vi "Examples - AcquisitionTest.vi"() -> ()   [LabVIEW 2018]
panel:
  in  "Stop":bool
  out "Image":T1(plugin-control)
  # "Use this button instead of Abort Execution button"
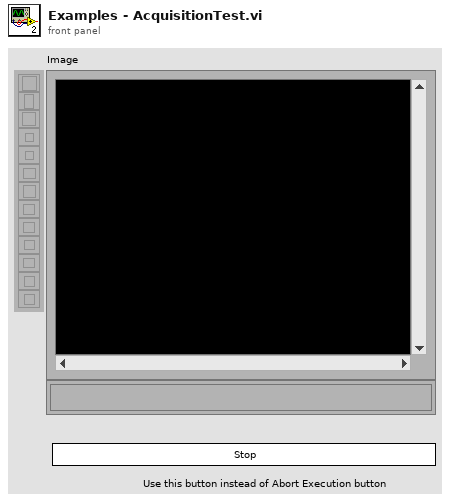
[diagram p1: front panel]
types:
  T1 = typedef "IMAQ Image.ctl" = refnum<image>
  T2 = typedef "Image Type" = u32
  T3 = typedef "xiImageMng - Attributes.ctl" = cluster{"WIDTH":i32, "HEIGHT":i32, "IMG_FORMAT":T4}
  T4 = typedef "IMG_DATA_FORMAT.ctl" = enum16{"MONO8", "MONO16", "RGB24", "RGB32", "RGBPLANAR", "RAW8", "RAW16"}
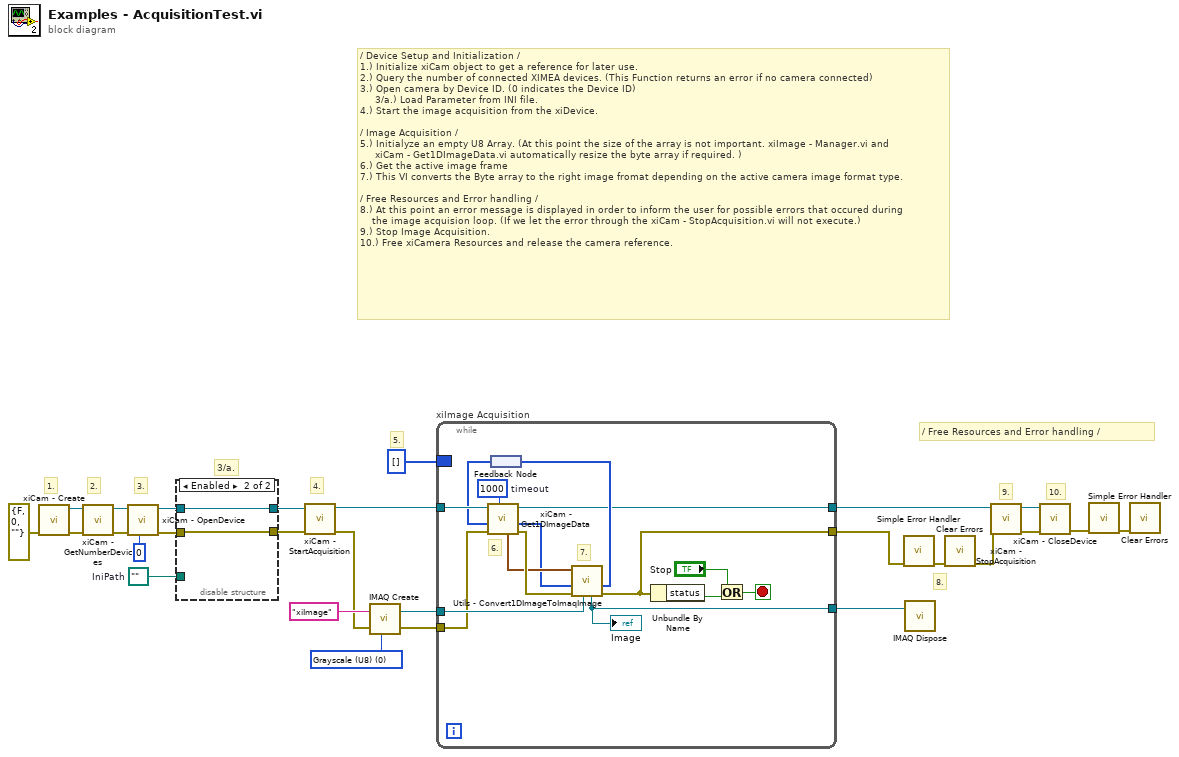
[diagram p0: block diagram]
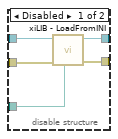
[diagram p2: hidden frame]
diagram:
  w4 = T2 0 items=["Grayscale (U8)", "Grayscale (I16)", "Grayscale (SGL)", "Complex (CSG)", "RGB (U32)", "HSL (U32)", "RGB (U64)", "Grayscale (U16)"] ("Image Type")
  w5 = path ""  # IniPath
  # "3/a."
  # "/ Free Resources and Error handling /"
  # "9."
  # "10."
  # "8."
  # "5."
  # "/ Device Setup and Initialization /\n1.) Initialize xiCam object to get a reference for later use.\n2.) Query the number of connected XIMEA devices. (This Function returns an error if no camera connected)\n3.) Open camera by Device ID. (0 indicates the Device ID)\n     3/a.) Load Parameter from INI file. \n4.) Start the image acquisition from the xiDevice.\n\n/ Image Acquisition /\n5.) Initialyze an empty U8 Array. (At this point the size of the array is not important. xiImage - Manager.vi and\n     xiCam - Get1DImageData.vi automatically resize the byte array if required. )\n6.) Get the active image frame\n7.) This VI converts the Byte array to the right image fromat depending on the active camera image format type.\n\n/ Free Resources and Error handling /\n8.) At this point an error message is displayed in order to inform the user for possible errors that occured during\n    the image acquision loop. (If we let the error through the xiCam - StopAcquisition.vi will not execute.)\n9.) Stop Image Acquisition.\n10.) Free xiCamera Resources and release the camera reference."
  # "4."
  # "3."
  # "2."
  # "1."
  n1 = call "xiCam - Create.vi"("error in (no error)"=errorcluster {"status"=FALSE, "code"=0, "source"=""}) -> ("error out"=w26:errorcluster, "new xiCam"=w27:refnum<k24>)  [unwired: 9 in]
  n2 = call "xiCam - GetNumberDevices.vi"("error in (no error)"=w26, "xiCam In"=w27) -> ("error out"=w24:errorcluster, "xiCam Out"=w25:refnum<k24>)  [unwired: 7 in, 1 out]
  n3 = call "xiCam - OpenDevice.vi"("DevID"=0, "error in (no error)"=w24, "xiCam In"=w25) -> ("error out"=w6:errorcluster, "xiCam Out"=w7:refnum<k24>)  [unwired: 7 in]
  n4 = disable-structure shown="Enabled" {
    disable-tunnel: w7 -> [w32 w34]
    disable-tunnel: [w31 w34] -> w3
    disable-tunnel: [w30 w33] -> w2
    disable-tunnel: w6 -> [w29 w33]
    disable-tunnel: w5 -> [w28 _]
    frame Disabled {
      n5 = call "xiLIB - LoadFromINI.vi"("IniPath"=w28, "Error In"=w29, "xiCam In"=w32) -> ("Error Out"=w30:errorcluster, "xiCam Out"=w31:refnum<k24>)  [unwired: 7 in]
    }
    frame Enabled {
    }
  }
  n6 = call "xiCam - StartAcquisition.vi"("error in (no error)"=w2, "xiCam In"=w3) -> ("error out"=w10:errorcluster, "xiCam Out"=w22:refnum<k24>)  [unwired: 8 in]
  n7 = call "IMAQ Create"("Image Name"="xiImage", "Image Type"=w4, "error in (no error)"=w10) -> ("New Image"=w11:T1, "error out"=w9:errorcluster)  [unwired: 2 in]
  n8 = while "xiImage Acquisition" {
    tunnel: w22 -> [w49]
    border: u8[] [] ("1DImageData Out") -> [_]
    tunnel: [w39] -> w19
    tunnel: [w38] -> w20
    tunnel: w11 -> [w37]
    tunnel: w9 -> [w36]
    tunnel: [w35] -> w8
    stop <- w40 stop-if-true
    w47 = 1000  # timeout
    # "7."
    # "6."
    n9 = feedback #1() -> (w48:u8[])
    n10 = call "xiCam - Get1DImageData.vi"("timeout"=w47, "error in (no error)"=w36, "1DImageData In"=w48, "xiCam In"=w49) -> ("error out"=w46:errorcluster, "1DImageData Out"=w44:u8[], "xiCam Out"=w38:refnum<k24>, "Image Properites"=w45:T3)  [unwired: 4 in]
    n11 = call "Utils - Convert1DImageToImaqImage.vi"("Image In"=w37, "error in (no error)"=w46, "1DImageData In"=w44, "Image Properties In"=w45) -> ("error out"=w39:errorcluster, "1DImageData Out"=w43:u8[], "Image Out"=w35:T1)  [unwired: 5 in]
    "Image" <- w35
    n12 = feedback-in #1(w43) -> ()
    n13 = Unbundle By Name(w39) -> ("status"=w42:bool)
    n14 = Or(x="Stop", y=w42) -> (x .or. y?=w40:bool)
  }
  n15 = call <vilib>:"Simple Error Handler.vi"("error in (no error)"=w19) -> ("error out"=w18:errorcluster)  [unwired: 4 in, 4 out]
  n16 = call "IMAQ Dispose"("Image"=w8) -> ()  [unwired: 5 in, 1 out]
  n17 = call <vilib>:"Clear Errors.vi"("error in (no error)"=w18) -> ("error out"=w17:errorcluster)  [unwired: 5 in, 1 out]
  n18 = call "xiCam - StopAcquisition.vi"("error in (no error)"=w17, "xiCam In"=w20) -> ("error out"=w15:errorcluster, "xiCam Out"=w16:refnum<k24>)  [unwired: 8 in]
  n19 = call "xiCam - CloseDevice.vi"("error in (no error)"=w15, "xiCam In"=w16) -> ("error out"=w13:errorcluster)  [unwired: 9 in]
  n20 = call <vilib>:"Simple Error Handler.vi"("error in (no error)"=w13) -> ("error out"=w14:errorcluster)  [unwired: 4 in, 4 out]
  n21 = call <vilib>:"Clear Errors.vi"("error in (no error)"=w14) -> ()  [unwired: 5 in, 2 out]
